vi "GetAlignmentVariables.vi"() -> ()   [LabVIEW 2018]
uses:
  AlignDUTVariables.vi
panel:
  in  "index":i32
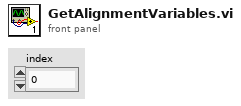
[diagram p1: front panel]
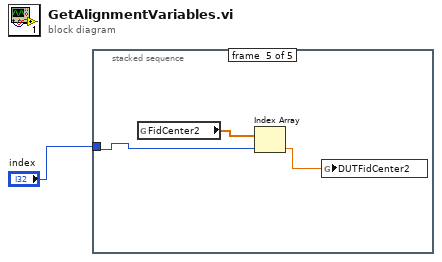
[diagram p0: block diagram]
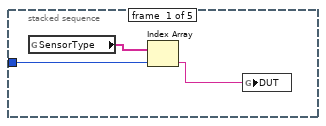
[diagram p2: hidden frame]
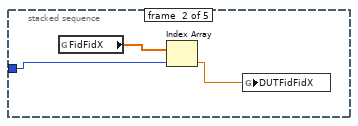
[diagram p3: hidden frame]
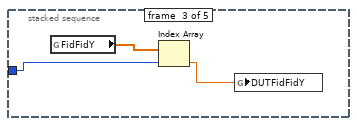
[diagram p4: hidden frame]
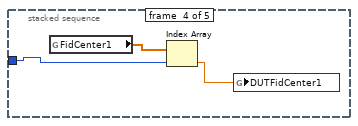
[diagram p5: hidden frame]
diagram:
  n1 = stacked-sequence {
    tunnel: "index" -> [w3 w5 w8 w11 w14]
    frame #0 {
      n2 = global read "AlignDUTVariables.vi" "SensorType"() -> (w4:string[])
      n3 = Index Array(array=w4, index=w3) -> (element=w2:string)
      n4 = global write "AlignDUTVariables.vi" "DUT"(w2) -> ()
    }
    frame #1 {
      n5 = global read "AlignDUTVariables.vi" "FidFidX"() -> (w6:dbl[])
      n6 = Index Array(array=w6, index=w5) -> (element=w7:dbl)
      n7 = global write "AlignDUTVariables.vi" "DUTFidFidX"(w7) -> ()
    }
    frame #2 {
      n8 = global read "AlignDUTVariables.vi" "FidFidY"() -> (w9:dbl[])
      n9 = Index Array(array=w9, index=w8) -> (element=w10:dbl)
      n10 = global write "AlignDUTVariables.vi" "DUTFidFidY"(w10) -> ()
    }
    frame #3 {
      n11 = global read "AlignDUTVariables.vi" "FidCenter1"() -> (w12:dbl[])
      n12 = Index Array(array=w12, index=w11) -> (element=w13:dbl)
      n13 = global write "AlignDUTVariables.vi" "DUTFidCenter1"(w13) -> ()
    }
    frame #4 {
      n14 = global read "AlignDUTVariables.vi" "FidCenter2"() -> (w15:dbl[])
      n15 = Index Array(array=w15, index=w14) -> (element=w16:dbl)
      n16 = global write "AlignDUTVariables.vi" "DUTFidCenter2"(w16) -> ()
    }
  }
